vi "_Update LC Out.vi"(5 "LC Stop":bool, 7 "LC Hold":bool) -> ()   [LabVIEW 2012]
uses:
  <vilib>/rvi/DataTransferAndStorage/Container/Common/niFpgaContainerGetUniqueNameForEmu.vi
  <vilib>/rvi/Memory/Memory_Emulation/niFpgaMemoryEmulationCacheClearOnFirstRun.vi
  <vilib>/rvi/Memory/Memory_Emulation/nirvimemoryEmulationManagerCache_MakeExclusive.vi
  <vilib>/rvi/Memory/Memory_Emulation/niFpgaMemoryEmulationValidateCache.vi
  <vilib>/rvi/Memory/Memory_Emulation/nirvimemoryEmulationManagerCache_ReleaseExclusive.vi
  <vilib>/rvi/Memory/Memory_Emulation/nirvimemoryEmulationManagerCache_InsertValue.vi
  <vilib>/Utility/error.llb/Clear Errors.vi
  <vilib>/rvi/Memory/Memory_Emulation/nirvimemoryEmulationManagerCache_GetValue.vi
  <vilib>/rvi/Emulation/niFpgaSctlEmulationGetInTimedLoop.vi
  <vilib>/rvi/Memory/Memory_Emulation/nirvimemoryEmulationManagerCache_SetValue.vi
  <vilib>/rvi/Emulation/niFpgaSctlEmulationResourceMgr.vi
  <vilib>/rvi/eio/common/nirviEmuTemplateMethod_errors.vi
  <vilib>/rvi/DataTransferAndStorage/Container/XNode/niFpgaContainer.xnode
  <vilib>/rvi/Memory/Memory_Emulation/nirvimemoryEmulation.vi
  <vilib>/eio/EIONode/EIONode.xnode
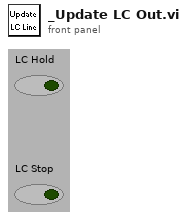
[diagram p1: front panel]
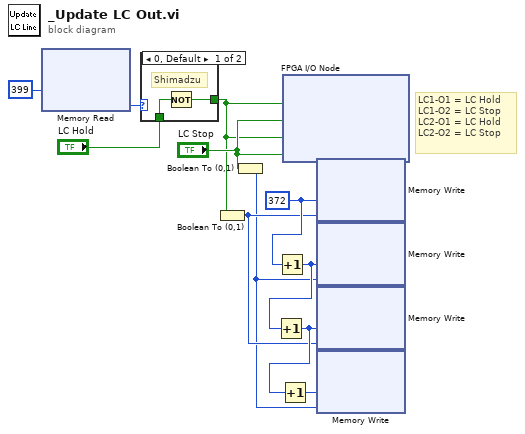
[diagram p0: block diagram]
diagram:
  w11 = u16 372 ("Address")
  # "LC1-O1 = LC Hold\nLC1-O2 = LC Stop\nLC2-O1 = LC Hold\nLC2-O2 = LC Stop"
  n1 = xnode ("Memory Read")("Address"=u16 399) -> ("Data"=w3:u32)  [unwired: 1 in, 1 out]
  n2 = case shown="0, Default" w3 {
    tunnel: "LC Hold" -> [w12 w14]
    tunnel: [w13 w14] -> w1
    frame 0, Default {
      # "Shimadzu"
      n3 = Not(x=w12) -> (.not. x?=w13:bool)
    }
    frame 1 {
      # "Other"
    }
  }
  n4 = Boolean To (0,1)(Boolean=w1) -> (0, 1=w6:i16)
  n5 = Boolean To (0,1)(Boolean="LC Stop") -> (0, 1=w5:i16)
  n6 = Increment(x=w11) -> (x+1=w10:u16)
  n7 = Increment(x=w10) -> (x+1=w8:u16)
  n8 = Increment(x=w8) -> (x+1=w9:u16)
  n9 = xnode "FPGA I/O Node"("Digtal IO/DIO49"=w1, "Digtal IO/DIO50"="LC Stop", "Digtal IO/DIO52"=w1, "Digtal IO/DIO56"="LC Stop") -> ()  [unwired: 4 in, 4 out]
  n10 = xnode ("Memory Write")("Address"=w11, "Data"=w6) -> ()  [unwired: 1 in, 1 out]
  n11 = xnode ("Memory Write")("Address"=w10, "Data"=w5) -> ()  [unwired: 1 in, 1 out]
  n12 = xnode ("Memory Write")("Address"=w8, "Data"=w6) -> ()  [unwired: 1 in, 1 out]
  n13 = xnode ("Memory Write")("Address"=w9, "Data"=w5) -> ()  [unwired: 1 in, 1 out]
